vi "GeraDados.vi"() -> ()   [LabVIEW 2017]
uses:
  <vilib>/Analysis/NI_AALBase.lvlib
panel:
  in  "SamplesPerGroup":i32=10
  out "String":string
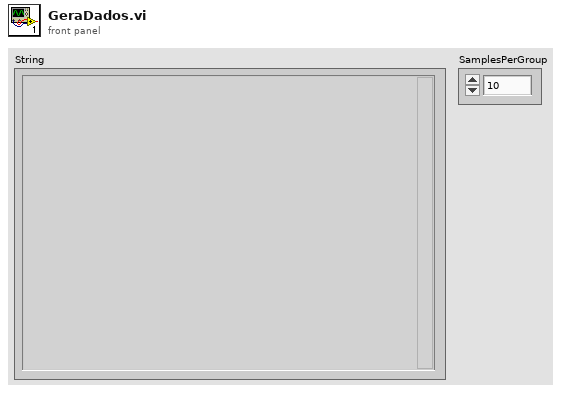
[diagram p1: front panel]
types:
  T1 = enum16{"open", "replace", "create", "open or create", "replace or create", "replace or create with confirmation"}
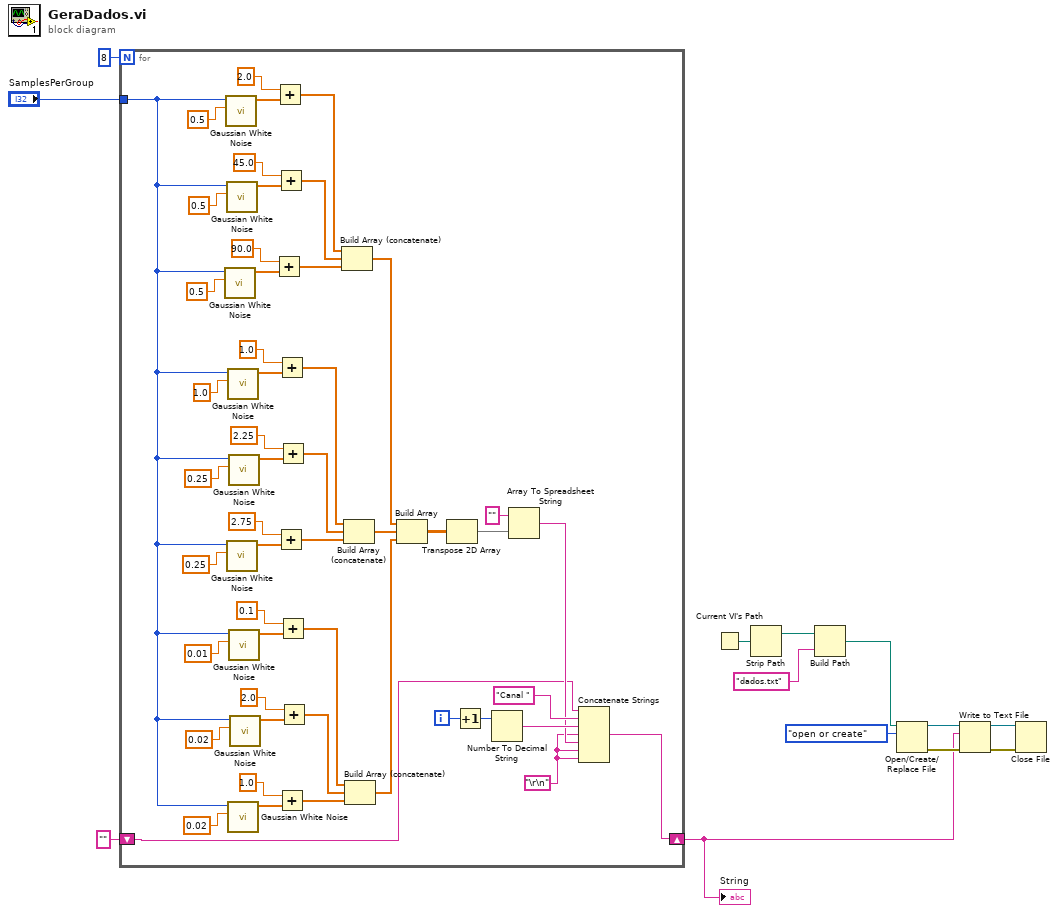
[diagram p0: block diagram]
diagram:
  n1 = for {
    N: 8 -> [_]
    shift-right: [w16] -> w3
    shift-left: "" -> [w15]
    tunnel: "SamplesPerGroup" -> [w14]
    i -> [w21]
    w17 = "\r\n"
    n2 = call <vilib>:"Gaussian White Noise.vi"("standard deviation"=0.5, "samples"=w14) -> ("Gaussian noise pattern"=w57:dbl[])  [unwired: 8 in, 1 out]
    n3 = call <vilib>:"Gaussian White Noise.vi"("standard deviation"=0.5, "samples"=w14) -> ("Gaussian noise pattern"=w63:dbl[])  [unwired: 8 in, 1 out]
    n4 = call <vilib>:"Gaussian White Noise.vi"("standard deviation"=0.5, "samples"=w14) -> ("Gaussian noise pattern"=w60:dbl[])  [unwired: 8 in, 1 out]
    n5 = call <vilib>:"Gaussian White Noise.vi"("standard deviation"=0.25, "samples"=w14) -> ("Gaussian noise pattern"=w48:dbl[])  [unwired: 8 in, 1 out]
    n6 = call <vilib>:"Gaussian White Noise.vi"("standard deviation"=1.0, "samples"=w14) -> ("Gaussian noise pattern"=w42:dbl[])  [unwired: 8 in, 1 out]
    n7 = call <vilib>:"Gaussian White Noise.vi"("standard deviation"=0.02, "samples"=w14) -> ("Gaussian noise pattern"=w33:dbl[])  [unwired: 8 in, 1 out]
    n8 = call <vilib>:"Gaussian White Noise.vi"("standard deviation"=0.25, "samples"=w14) -> ("Gaussian noise pattern"=w45:dbl[])  [unwired: 8 in, 1 out]
    n9 = call <vilib>:"Gaussian White Noise.vi"("standard deviation"=0.01, "samples"=w14) -> ("Gaussian noise pattern"=w39:dbl[])  [unwired: 8 in, 1 out]
    n10 = call <vilib>:"Gaussian White Noise.vi"("standard deviation"=0.02, "samples"=w14) -> ("Gaussian noise pattern"=w36:dbl[])  [unwired: 8 in, 1 out]
    n11 = Add(x=90.0 ("standard deviation"), y=w57) -> (x+y=w53:dbl[])
    n12 = Add(x=2.0 ("standard deviation"), y=w63) -> (x+y=w55:dbl[])
    n13 = Add(x=45.0 ("standard deviation"), y=w60) -> (x+y=w54:dbl[])
    n14 = Add(x=2.75 ("standard deviation"), y=w48) -> (x+y=w52:dbl[])
    n15 = Add(x=1.0 ("standard deviation"), y=w42) -> (x+y=w50:dbl[])
    n16 = Add(x=1.0 ("standard deviation"), y=w33) -> (x+y=w29:dbl[])
    n17 = Add(x=2.25 ("standard deviation"), y=w45) -> (x+y=w51:dbl[])
    n18 = Add(x=0.1 ("standard deviation"), y=w39) -> (x+y=w31:dbl[])
    n19 = Add(x=2.0 ("standard deviation"), y=w36) -> (x+y=w30:dbl[])
    n20 = Build Array (concatenate)(w55, w54, w53) -> (w27:dbl[])
    n21 = Build Array (concatenate)(w50, w51, w52) -> (w28:dbl[])
    n22 = Build Array (concatenate)(w31, w30, w29) -> (w26:dbl[])
    n23 = Build Array(w27, w28, w26) -> (w25:dbl[][])
    n24 = Transpose 2D Array(2D array=w25) -> (transposed array=w24:dbl[][])
    n25 = Increment(x=w21) -> (x+1=w22:i32)
    n26 = Number To Decimal String(number=w22) -> (decimal integer string=w20:string)  [unwired: 1 in]
    n27 = Array To Spreadsheet String(array=w24, 3:"" ("format string")) -> (spreadsheet string=w18:string)  [unwired: 1 in]
    n28 = Concatenate Strings(w15, "Canal " ("string"), w20, w17, w18, w17, w17) -> (w16:string)
  }
  "String" <- w3
  n29 = Current VI's Path() -> (path=w9:path)
  n30 = Strip Path(path=w9) -> (stripped path=w8:path)  [unwired: 1 out]
  n31 = Build Path(base path=w8, name or relative path="dados.txt") -> (appended path=w6:path)
  n32 = Open/Create/Replace File(file path (use dialog)=w6, operation (0:open)=T1."open or create") -> (refnum out=w4:refnum<file>, error out=w5:errorcluster)  [unwired: 4 in, 1 out]
  n33 = Write to Text File(file (use dialog)=w4, text=w3, error in=w5) -> (refnum out=w1:refnum<file>, error out=w2:errorcluster)  [unwired: 1 in, 1 out]
  n34 = Close File(refnum=w1, error in=w2) -> ()  [unwired: 2 out]
